vi "Configure Control AO Range.vi"(0 "VISA resource name":refnum<visa-resource-name>, 1 "Scaling Lower Limit":i32=-270, 2 "Term. No.(0:OUT1)":u16(ring) items=["OUT1", "PV1", "SP1", "OUT2", "PV2", "SP2"], 5 "Unit No. (0)":i32 min=0 max=6, 7 "Module No.(0)":i32 min=0 max=9, 9 "AO No.(1)":i32=1 min=1 max=2, 11 "error in (no error)":errorcluster, 12 "Trans. Out(false)":bool, 13 "Scaling Upper Limit":i32=1370) -> (4 "VISA resource name out":refnum<visa-resource-name>, 6 "AO No.":i32, 8 "Unit No.":i32, 10 "Module No.":i32, 15 "error out":errorcluster)   [LabVIEW 2020, in "Yokogawa GX Series.lvlib"]
doc: "Set AO Range of PID module.\n\nCommand: SCtrlRangeAO"
uses:
  <instrlib>/Yokogawa GX Series/Yokogawa GX Series.lvlib
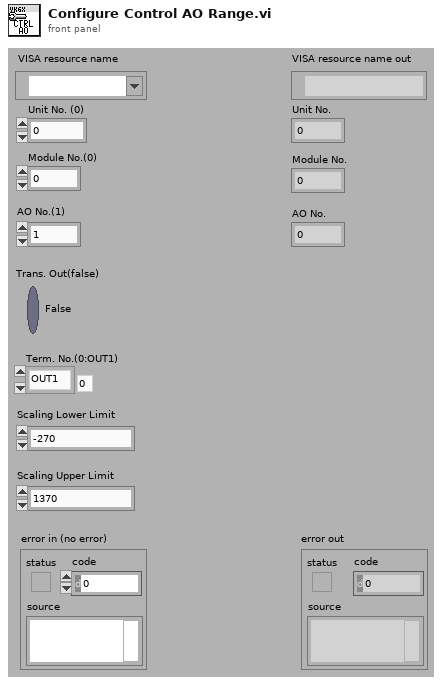
[diagram p1: front panel]
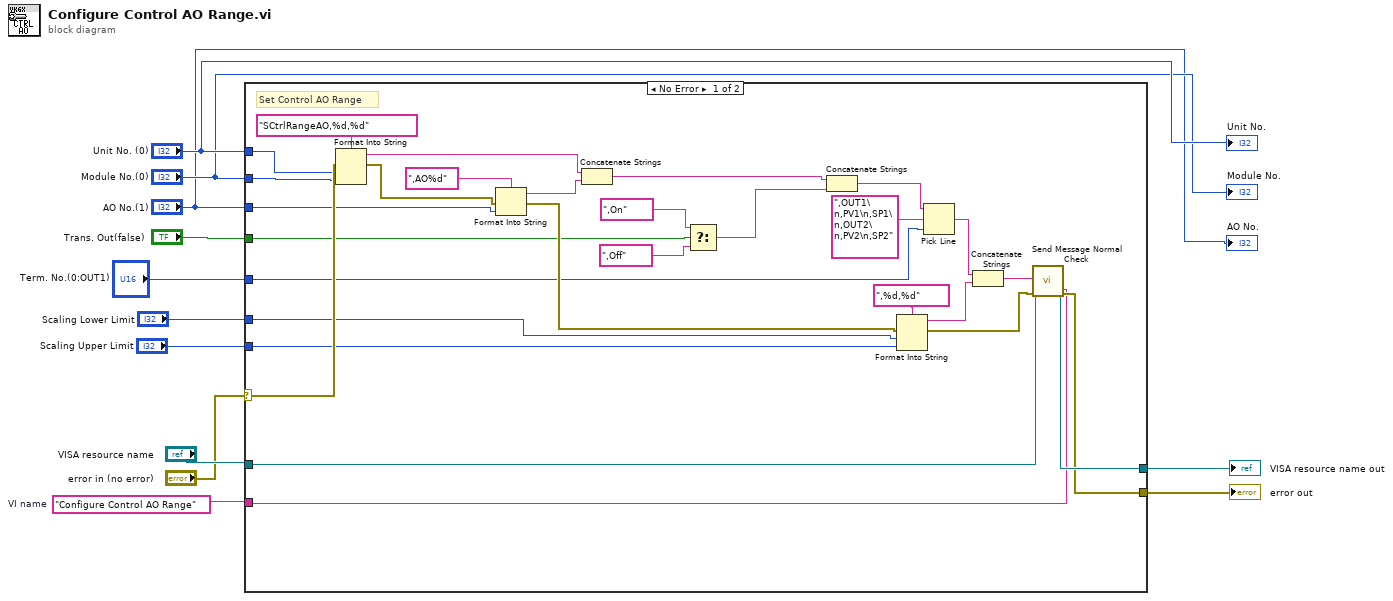
[diagram p0: block diagram]
diagram:
  w8 = "Configure Control AO Range"  # VI name
  n1 = case shown="No Error" "error in (no error)" {
    selector: "error in (no error)" -> [w37 w42]
    tunnel: [w41 w43] -> w12
    tunnel: [w40 w42] -> w11
    tunnel: "VISA resource name" -> [w39 w43]
    tunnel: w8 -> [w36 _]
    tunnel: "Unit No. (0)" -> [w35 _]
    tunnel: "Module No.(0)" -> [w34 _]
    tunnel: "AO No.(1)" -> [w32 _]
    tunnel: "Scaling Lower Limit" -> [w14 _]
    tunnel: "Trans. Out(false)" -> [w18 _]
    tunnel: "Scaling Upper Limit" -> [w13 _]
    tunnel: "Term. No.(0:OUT1)" -> [w19 _]
    frame No Error {
      # "Set Control AO Range"
      n2 = Format Into String(format string="SCtrlRangeAO,%d,%d", error in=w37, w35, w34) -> (resulting string=w30:string, error out=w31:errorcluster)  [unwired: 1 in]
      n3 = Format Into String(format string=",AO%d", error in=w31, w32) -> (resulting string=w29:string, error out=w21:errorcluster)  [unwired: 1 in]
      n4 = Concatenate Strings(w30, w29) -> (w23:string)
      n5 = Select(t=",On", s=w18, f=",Off") -> (s? t:f=w15:string)
      n6 = Concatenate Strings(w23, w15) -> (w26:string)
      n7 = Format Into String(format string=",%d,%d", error in=w21, w14, w13) -> (resulting string=w27:string, error out=w20:errorcluster)  [unwired: 1 in]
      n8 = Pick Line(string ("")=w26, multi-line string=",OUT1\n,PV1\n,SP1\n,OUT2\n,PV2\n,SP2", line index=w19) -> (output string=w24:string)
      n9 = Concatenate Strings(w24, w27) -> (w22:string)
      n10 = call <instrlib>:"Send Message Normal Check.vi"("Source (\"\")"=w36, "error in (no error)"=w20, "Send Message (\"\")"=w22, "VISA resource name"=w39) -> ("error out"=w40:errorcluster, "VISA resource name out"=w41:refnum<visa-resource-name>)  [unwired: 2 in, 4 out]
    }
    frame Error {
    }
  }
  "error out" <- w11
  "VISA resource name out" <- w12
  "Unit No." <- "Unit No. (0)"
  "Module No." <- "Module No.(0)"
  "AO No." <- "AO No.(1)"
